vi "distribute_setpoints.vi"(8 "setpoints":dbl[](array[numeric]), 9 "Magnitude":dbl, 10 "Angle":dbl, 11 "Frequency":dbl) -> (2 "references":T1)   [LabVIEW 2021]
uses:
  General Purpose/references.ctl
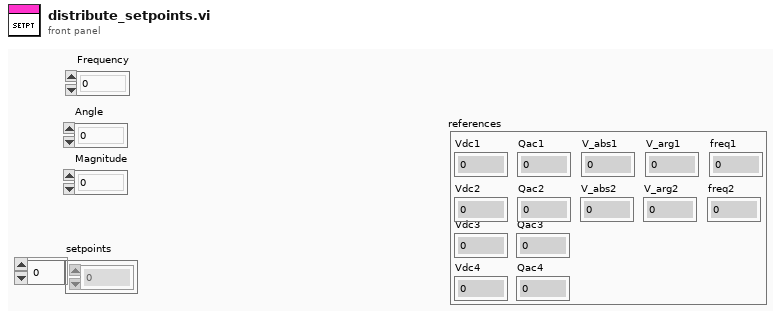
[diagram p1: front panel]
types:
  T1 = typedef "references.ctl" = cluster{"Vdc1":dbl, "Vdc2":dbl, "Qac2":dbl, "Vdc3":dbl, "Qac3":dbl, "Vdc4":dbl, "Qac4":dbl, "Qac1":dbl, "V_arg2":dbl, "V_abs2":dbl, "V_abs1":dbl, "V_arg1":dbl, "freq1":dbl, "freq2":dbl}
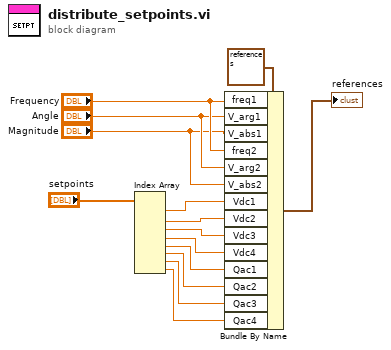
[diagram p0: block diagram]
diagram:
  n1 = Index Array(array="setpoints") -> (element #1=w9:dbl, element #2=w7:dbl, element #3=w6:dbl, element #4=w5:dbl, element #5=w4:dbl, element #6=w3:dbl, element #7=w2:dbl, element #8=w1:dbl)  [unwired: 8 in]
  n2 = Bundle By Name(cluster=T1 {"Vdc1"=0.0, "Vdc2"=0.0, "Qac2"=0.0, "Vdc3"=0.0, "Qac3"=0.0, "Vdc4"=0.0, "Qac4"=0.0, "Qac1"=0.0, "V_arg2"=0.0, "V_abs2"=0.0, "V_abs1"=0.0, "V_arg1"=0.0, "freq1"=0.0, "freq2"=0.0} ("references 2"), "freq1"="Frequency", "V_arg1"="Angle", "V_abs1"="Magnitude", "freq2"="Frequency", "V_arg2"="Angle", "V_abs2"="Magnitude", "Vdc1"=w9, "Vdc2"=w7, "Vdc3"=w6, "Vdc4"=w5, "Qac1"=w4, "Qac2"=w3, "Qac3"=w2, "Qac4"=w1) -> (→"references":T1)
